vi "programa 6 control2.vi"() -> ()   [LabVIEW 2011]
uses:
  Control2.ctl
  <vilib>/express/express arith-compare/Formula/XNode/ExpressFormulaBlockNode.xnode
panel:
  out "Array 2":string[](array[string])
  out "Array":dbl[](array[numeric])
  # "En el arreglo 1 ingresar 5 numeros enteros y luego en el arreglo 2\nescribir si es par o impar cada uno de los numeros."
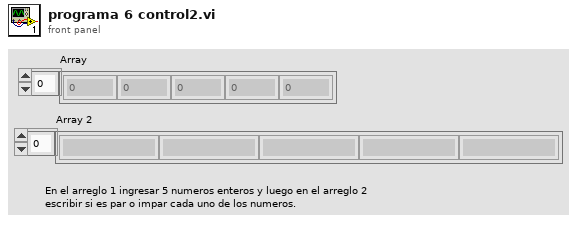
[diagram p1: front panel]
types:
  T1 = typedef "Control2.ctl" = enum16{"iniciar arreglos", "rellenar arreglo1", "encontrarPareImpar", "final"}
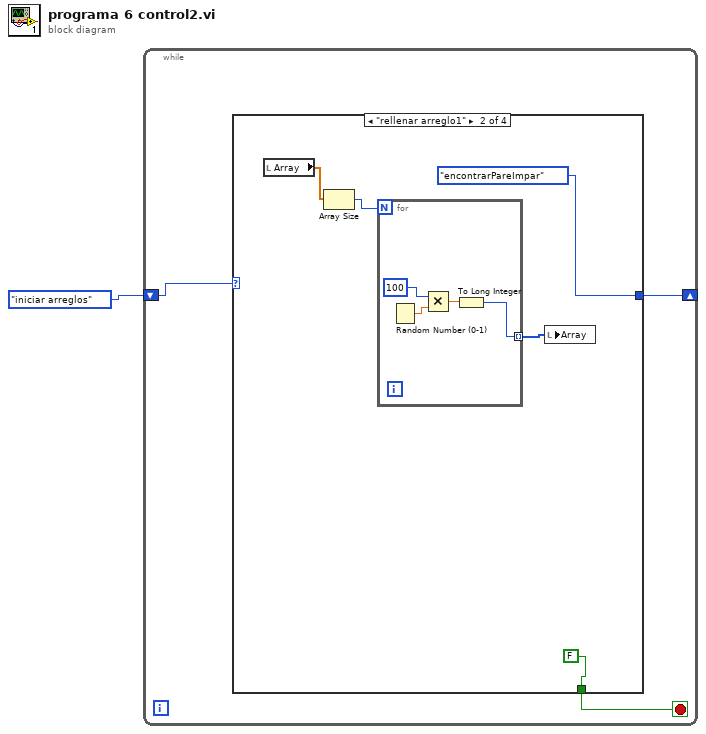
[diagram p0: block diagram]
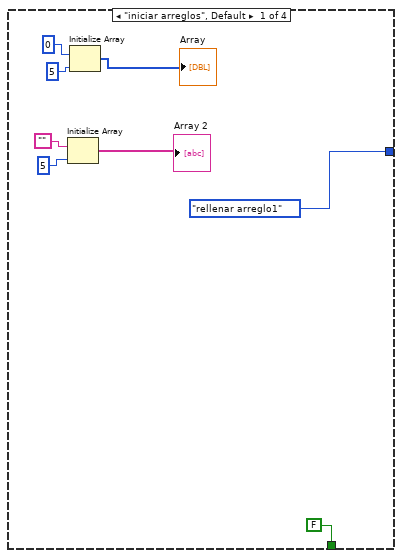
[diagram p2: hidden frame]
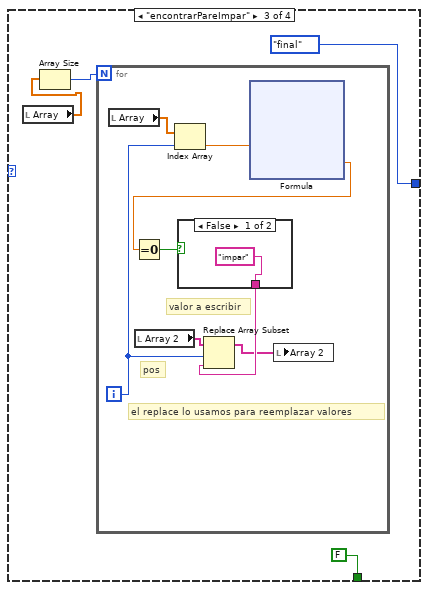
[diagram p3: hidden frame]
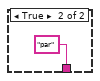
[diagram p4: hidden frame]
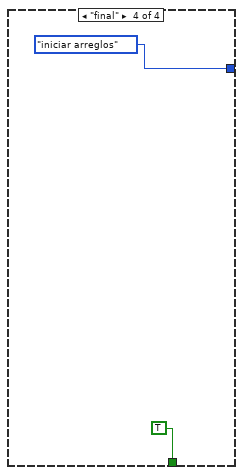
[diagram p5: hidden frame]
diagram:
  n1 = while {
    shift-right: [w3] -> _
    shift-left: Control2."iniciar arreglos" -> [w4]
    stop <- w2 stop-if-true
    n2 = case shown="\"rellenar arreglo1\"" w4 {
      tunnel: [Control2."rellenar arreglo1" Control2."encontrarPareImpar" Control2."final" Control2."iniciar arreglos"] -> w3
      tunnel: [FALSE FALSE FALSE TRUE] -> w2
      frame "iniciar arreglos", Default {
        n3 = Initialize Array "Initialize Array"("", 5) -> (→"Array 2":string[])
        n4 = Initialize Array "Initialize Array"(0, 5) -> (→"Array":i32[])
      }
      frame "rellenar arreglo1" {
        n5 = local read "Array"() -> (w17:dbl[])
        n6 = Array Size(array=w17) -> (size(s)=w13:i32)
        n7 = for {
          N: w13 -> [_]
          tunnel: [w18] -> w16 mode=indexing
          n8 = Random Number (0-1)() -> (number: 0 to 1=w20:dbl)
          n9 = Multiply(x=100, y=w20) -> (x*y=w19:dbl)
          n10 = To Long Integer(number=w19) -> (32bit integer=w18:i32)
        }
        n11 = local write "Array"(w16) -> ()
      }
      frame "encontrarPareImpar" {
        n12 = local read "Array"() -> (w24:dbl[])
        n13 = Array Size(array=w24) -> (size(s)=w25:i32)
        n14 = for {
          N: w25 -> [_]
          i -> [w28]
          # "el replace lo usamos para reemplazar valores"
          # "pos"
          # "valor a escribir"
          n15 = local read "Array"() -> (w33:dbl[])
          n16 = local read "Array 2"() -> (w29:string[])
          n17 = Index Array "Index Array"(array=w33, index=w28) -> (element=w32:dbl)
          n18 = xnode "Formula"("X1"=w32) -> ("Result"=w31:dbl)  [unwired: 1 in, 1 out]
          n19 = Equal To 0?(x=w31) -> (x = 0?=w30:bool)
          n20 = case shown="False" w30 {
            tunnel: ["impar" "par"] -> w27
            frame False {
            }
            frame True {
            }
          }
          n21 = Replace Array Subset "Replace Array Subset"(array=w29, new element=w27, index=w28) -> (w26:string[])
          n22 = local write "Array 2"(w26) -> ()
        }
      }
      frame "final" {
      }
    }
  }
